vi "KRASS Hiport_timing engineer.vi"(8 "error in (no error)":errorcluster, 9 "WaitTime":dbl, 11 "VISA resource name":refnum<visa-resource-name>) -> (0 "error in (no error) 2":errorcluster, 1 "Result":bool, 2 "Report":string, 3 "VISA resource name out":refnum<visa-resource-name>)   [LabVIEW 2015]
panel:
  out "String":string
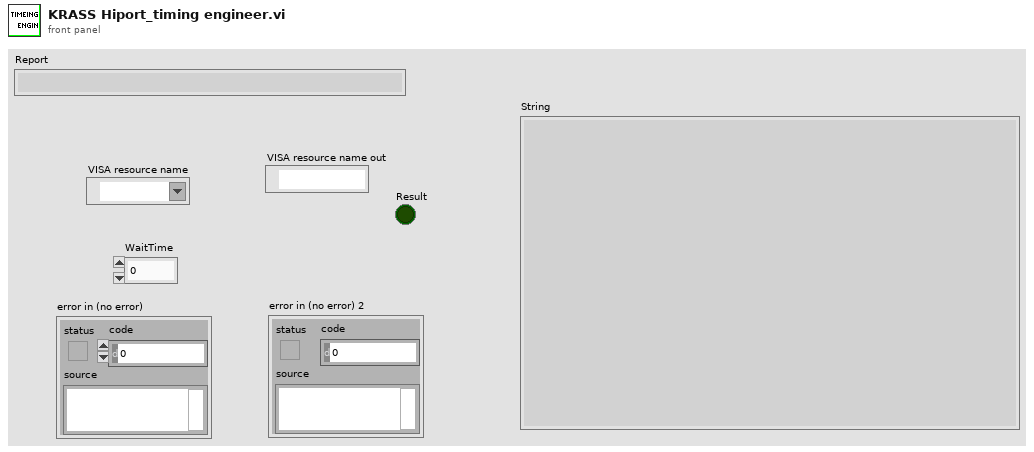
[diagram p1: front panel]
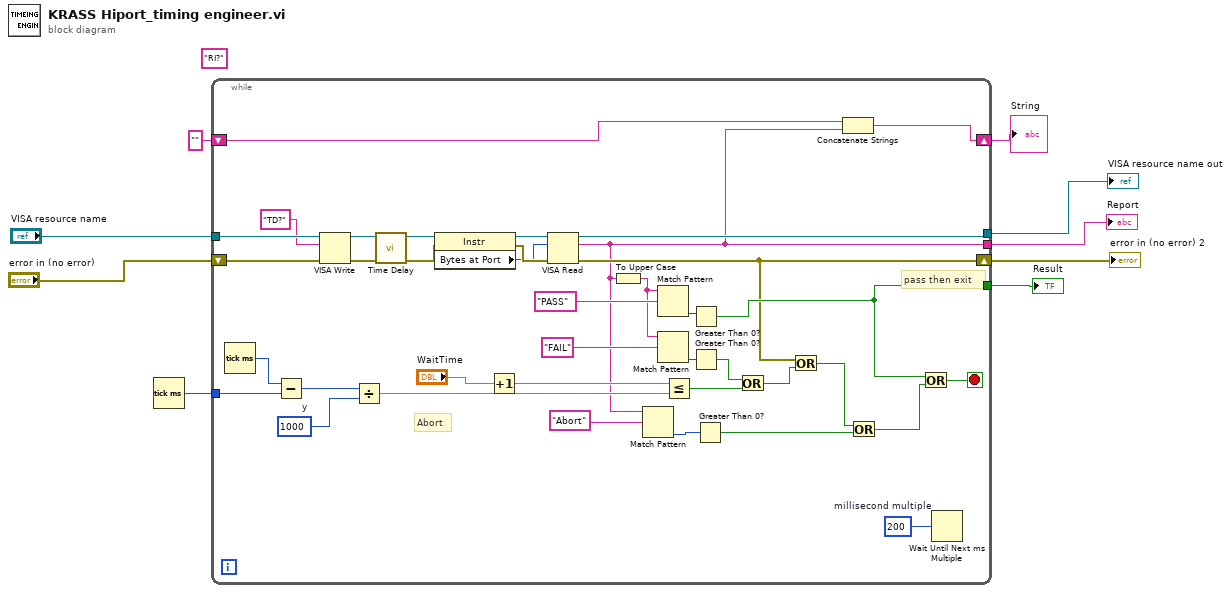
[diagram p0: block diagram]
diagram:
  (unwired) "RI?"
  n1 = Tick Count (ms)() -> (millisecond timer value=w9:u32)
  n2 = while {
    tunnel: w9 -> [w45]
    tunnel: "VISA resource name" -> [w35]
    shift-right: [w16] -> w6
    shift-left: "error in (no error)" -> [w29]
    tunnel: [w11] -> w5
    tunnel: [w27] -> w4
    tunnel: [w20] -> w3
    shift-right: [w13] -> w1
    shift-left: "" -> [w12]
    stop <- w30 stop-if-true
    w28 = u32 200  # millisecond multiple
    w43 = u32 1000  # y
    # "Abort"
    # "pass then exit"
    n3 = Tick Count (ms)() -> (millisecond timer value=w46:u32)
    n4 = Subtract(x=w46, y=w45) -> (x-y=w44:u32)
    n5 = VISA Write(VISA resource name=w35, write buffer="TD?", error in (no error)=w29) -> (VISA resource name out=w41:refnum<visa-resource-name>, error out=w40:errorcluster)  [unwired: 1 out]
    n6 = Divide(x=w44, y=w43) -> (x/y=w26:dbl)
    n7 = call "Time Delay"("error in (no error)"=w40) -> ("error out"=w39:errorcluster)  [unwired: 10 in]
    n8 = property class="Instr"(reference=w41, error in=w39) -> (reference out=w38:refnum<visa-resource-name>, error out=w37:errorcluster, "Bytes at Port"=w36:u32)
    n9 = Increment(x="WaitTime") -> (x+1=w25:dbl)
    n10 = VISA Read(VISA resource name=w38, byte count=w36, error in (no error)=w37) -> (VISA resource name out=w27:refnum<visa-resource-name>, read buffer=w11:string, error out=w16:errorcluster)  [unwired: 1 out]
    n11 = To Upper Case(1:w11) -> (0:w21:string)
    n12 = Match Pattern(string=w11, regular expression="Abort") -> (offset past match=w18:i32)  [unwired: 1 in, 3 out]
    n13 = Match Pattern(string=w21, regular expression="PASS") -> (offset past match=w33:i32)  [unwired: 1 in, 3 out]
    n14 = Match Pattern(string=w21, regular expression="FAIL") -> (offset past match=w23:i32)  [unwired: 1 in, 3 out]
    n15 = Less Or Equal?(x=w25, y=w26) -> (x <= y?=w31:bool)
    n16 = Greater Than 0?(x=w33) -> (x > 0?=w20:bool)
    n17 = Greater Than 0?(x=w23) -> (x > 0?=w22:bool)
    n18 = Greater Than 0?(x=w18) -> (x > 0?=w17:bool)
    n19 = Or(x=w22, y=w31) -> (x .or. y?=w15:bool)
    n20 = Or(x=w16, y=w15) -> (x .or. y?=w14:bool)
    n21 = Concatenate Strings(w12, w11) -> (w13:string)
    n22 = Or(x=w14, y=w17) -> (x .or. y?=w10:bool)
    n23 = Or(x=w20, y=w10) -> (x .or. y?=w30:bool)
    n24 = Wait Until Next ms Multiple(millisecond multiple=w28) -> ()  [unwired: 1 out]
  }
  "error in (no error) 2" <- w6
  "Report" <- w5
  "VISA resource name out" <- w4
  "Result" <- w3
  "String" <- w1
